vi "Claw Rotation Controller.vi"(8 "error in":errorcluster) -> ()   [LabVIEW 2017]
doc: "This VI executes continuously carrying out the current operation and responding to updates or new operations. It will often contain the timing or control code that is difficult to place directly in TeleOp. This VI generally opens all sensors and motors and isolates the rest of the robot code from knowing how the operations are carried out."
uses:
  Claw Rotation Setpoints.ctl
  Claw Rotation Operations.ctl
  Users/Public/Documents/Cross The Road Electronics/Phoenix-LabVIEW/Motor Controller/Controls/CTRE_Phoenix_MotorControl_ControlMode.ctl
  <vilib>/Rock Robotics/WPI/ThirdParty/Phoenix-LabVIEW/Motor Controller/Controls/CTRE_Phoenix_MotorControl_NeutralMode.ctl
  <vilib>/Rock Robotics/SystemInterfaces/DIO/FPGA_DIOChannel.ctl
  <vilib>/addons/control/pid/pid.llb/PID (DBL).vi
  <vilib>/addons/control/pid/NI_PID_pid.lvlib
  <vilib>/Rock Robotics/Network Tables/NT Write Boolean.vi
panel:
  out "Current\nCmd":string
  # "Tip: It may be helpful to observe inputs and sensor values.\nYou may also want to display tuning or debugging controls."
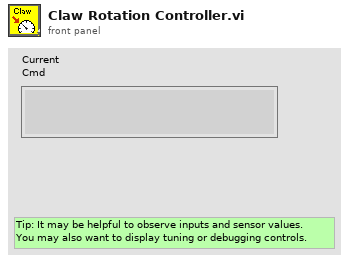
[diagram p1: front panel]
types:
  T1 = typedef "FPGA_DIOChannel.ctl" = enum8{"DIO 0", "DIO 1", "DIO 2", "DIO 3", "DIO 4", "DIO 5", "DIO 6", "DIO 7", "DIO 8", "DIO 9", "DIO MXP 0", "DIO MXP 1", "DIO MXP 2", "DIO MXP 3", "DIO MXP 4", "DIO MXP 5", "DIO MXP 6", "DIO MXP 7", "DIO MXP 8", "DIO MXP 9", "DIO MXP 10", "DIO MXP 11", "DIO MXP 12", "DIO MXP 13", "DIO MXP 14", "DIO MXP 15", "SPI Port CS1", "SPI Port CS2", "SPI Port CS3", "SPI Port MISO", "SPI Port MOSI", "Invalid"}
  T2 = typedef "CTRE_Phoenix_MotorControl_ControlMode.ctl" = u16
  T3 = typedef "CTRE_Phoenix_MotorControl_NeutralMode.ctl" = enum8{"EEPROMSetting", "Override to Coast", "Override to Brake"}
  T4 = typedef "Claw Rotation Setpoints.ctl" = cluster{"Operation":T5, "Setpoint":dbl, "Duration":dbl}
  T5 = typedef "Claw Rotation Operations.ctl" = enum16{"Reserve", "Read Current", "Immediate", "Rotate Manual", "Preset Position"}
  T6 = typedef "WPI_MotorControlDeviceRef.ctl" = cluster{"DeviceStatus":errorcluster, "Type":T7, "PWM":cluster{"PWM Channel":T8, "DeadBand":T9}, "CAN":cluster{"Device Number":u8, "SetOutput VI Ref":variant, "GetOutput VI Ref":variant, "Enable VI Ref":variant, "Disable VI Ref":variant, "Data":variant}, "Invert":bool, "DIO PWM":cluster{"PWM \"Enable\" Channel":T8, "DIOChannel":T1, "PWM Rate":dbl}}
  T7 = typedef "WPI_MotorControlType.ctl" = enum16{"PWM", "CAN", "DIO PWM"}
  T8 = typedef "FPGA_DIOPWMChannel.ctl" = enum8{"PWM 0", "PWM 1", "PWM 2", "PWM 3", "PWM 4", "PWM 5", "PWM 6", "PWM 7", "PWM 8", "PWM 9", "PWM MXP 0", "PWM MXP 1", "PWM MXP 2", "PWM MXP 3", "PWM MXP 4", "PWM MXP 5", "PWM MXP 6", "PWM MXP 7", "PWM MXP 8", "PWM MXP 9", "Invalid"}
  T9 = typedef "WPI_PWMDeadband.ctl" = cluster{"Name":string, "maxPositivePwm":i32, "minPositivePwm":i32, "centerPwm":i32, "maxNegativePwm":i32, "minNegativePwm":i32, "angularRange":u16}
  T10 = typedef "WPI_DigitalInputDevRef.ctl" = cluster{"DevStatus":errorcluster, "DIO Channel":T1}
  T11 = typedef "Command Status Info.ctl" = cluster{"Name":string, "Status":T12, "notifier out":T13}
  T12 = typedef "Completion Status.ctl" = enum16{"Successful", "Aborted", "Incomplete"}
  T13 = typedef "Completion Notifier.ctl" = refnum<notifier>
  T14 = cluster{"Current Command":T4, "Command Timing":cluster{"Start Time (ms)":u32, "Iterations":i32}, "Command Arguments":cluster{"Command Info":T11, "Description":string, "Default Command":T4, "queue out":refnum<queue>, "Subsystem Name":string}}
  T15 = cluster{"proportional gain (Kc)":dbl, "integral time (Ti, min)":dbl, "derivative time (Td, min)":dbl}
  T16 = typedef "WPI_AnalogChannelDevRef.ctl" = cluster{"DevStatus":errorcluster, "Analog Channel":T17}
  T17 = typedef "FPGA_AIChannel.ctl" = enum8{"AI 0", "AI 1", "AI 2", "AI 3", "AI MXP 0", "AI MXP 1", "AI MXP 2", "AI MXP 3", "Invalid"}
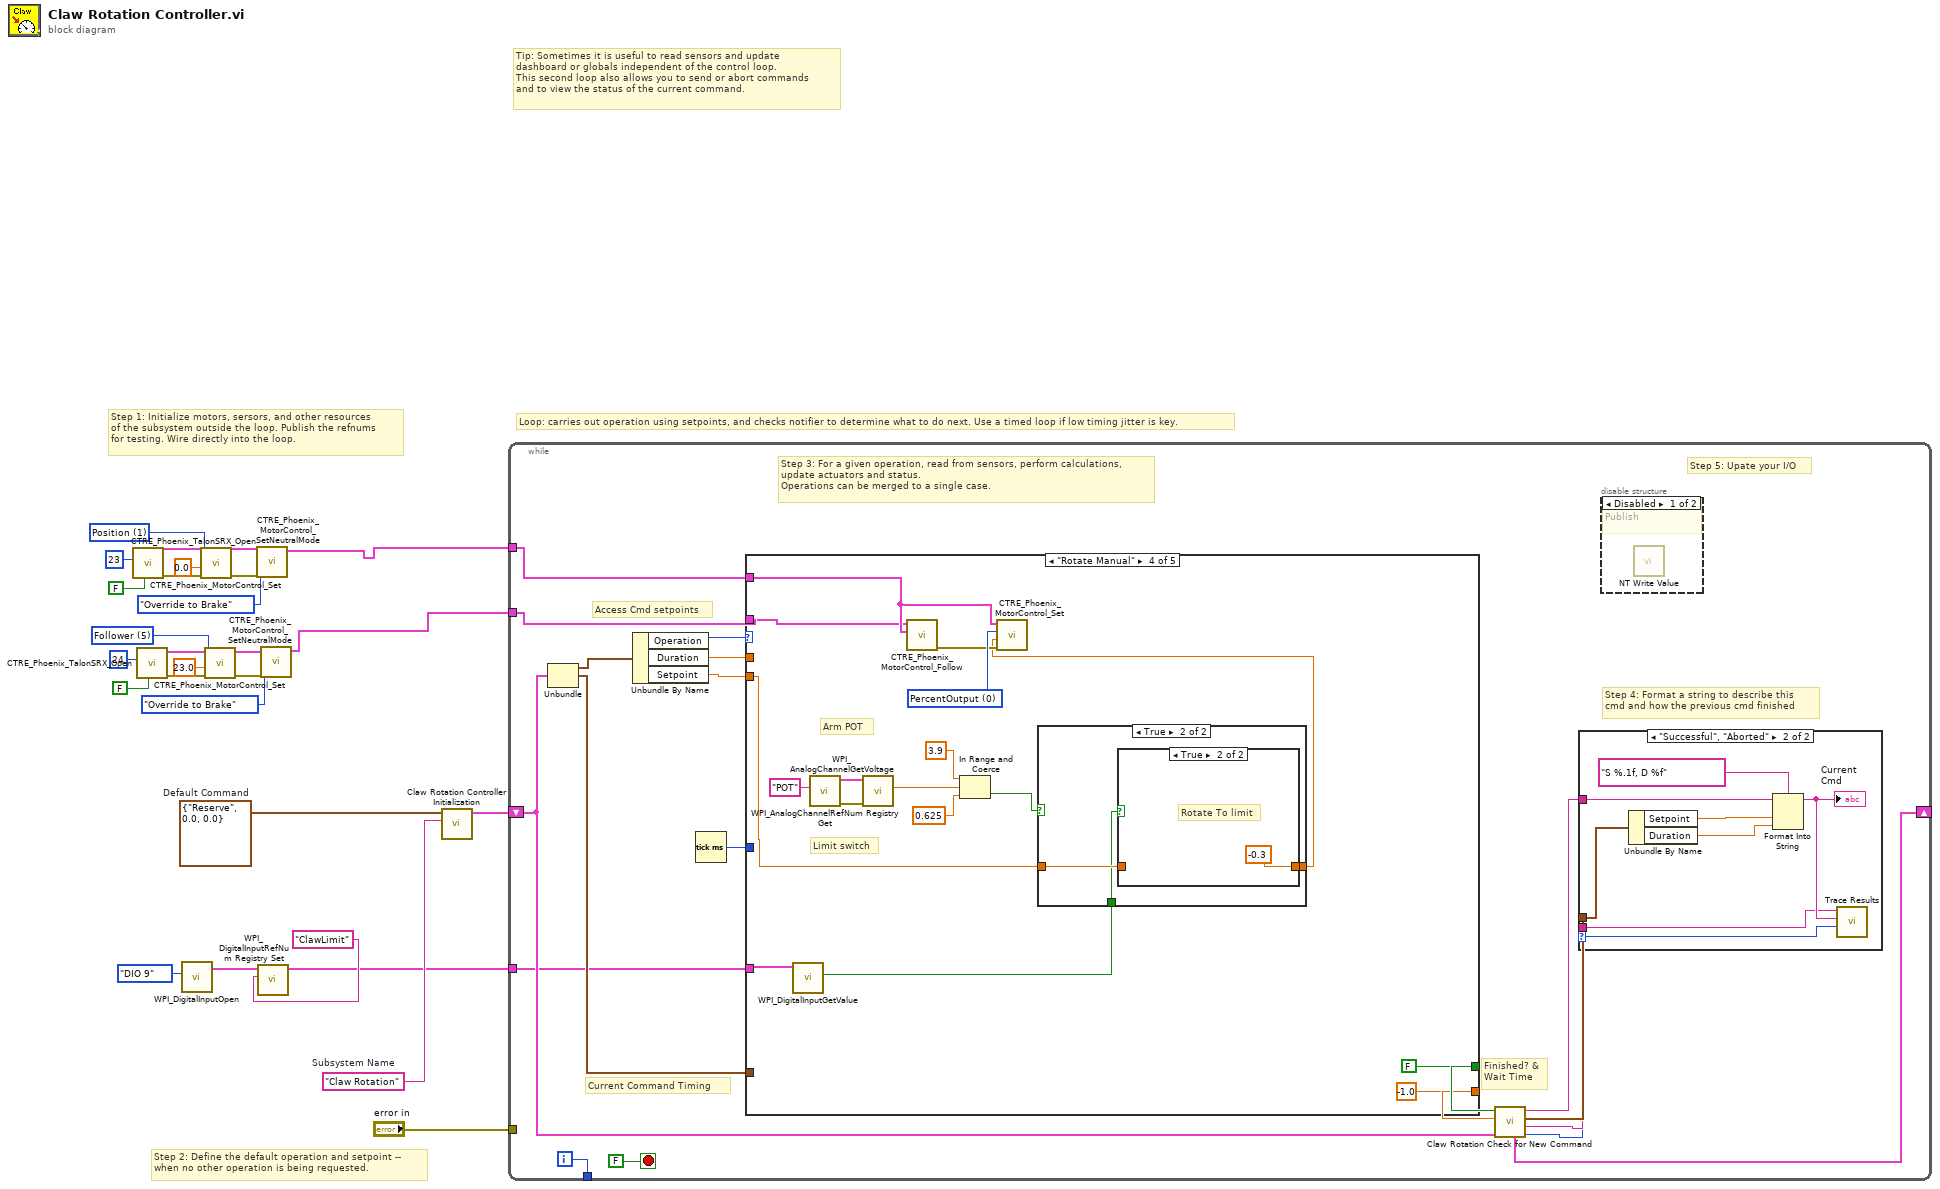
[diagram p0: block diagram]
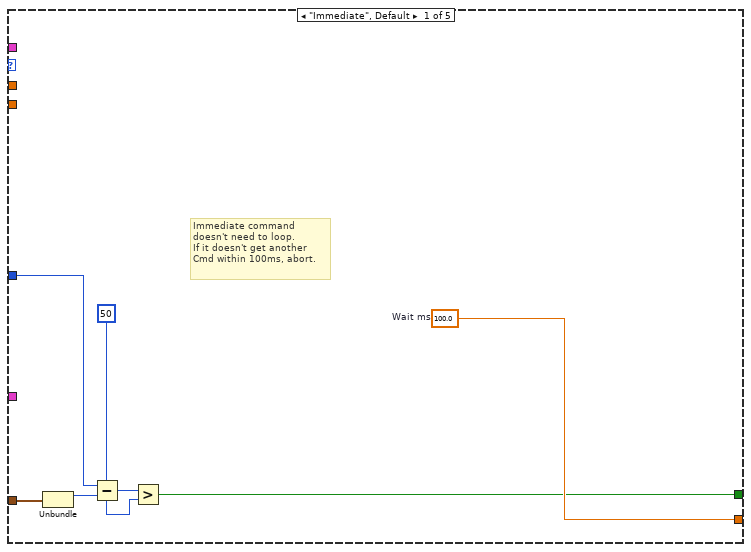
[diagram p4: hidden frame]
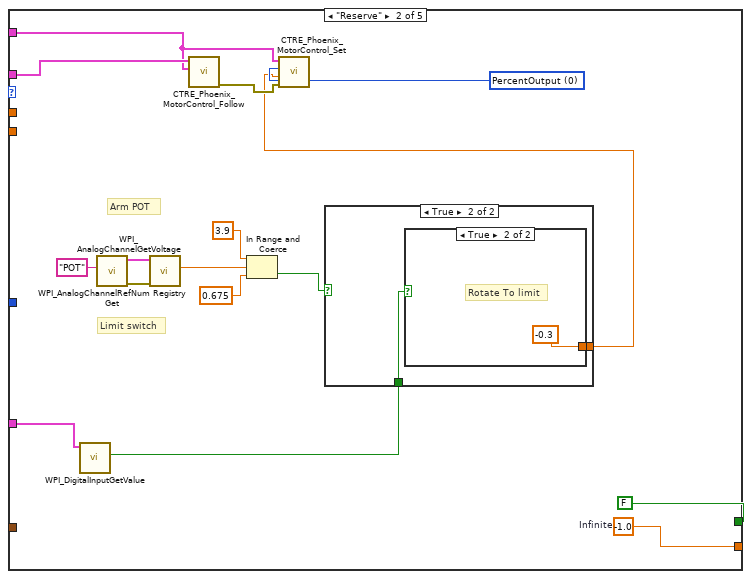
[diagram p5: hidden frame]
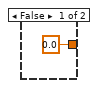
[diagram p6: hidden frame]
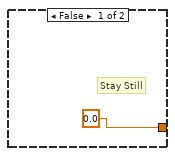
[diagram p7: hidden frame]
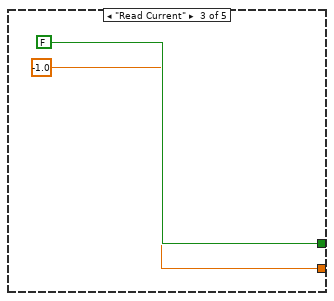
[diagram p8: hidden frame]
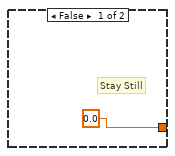
[diagram p10: hidden frame]
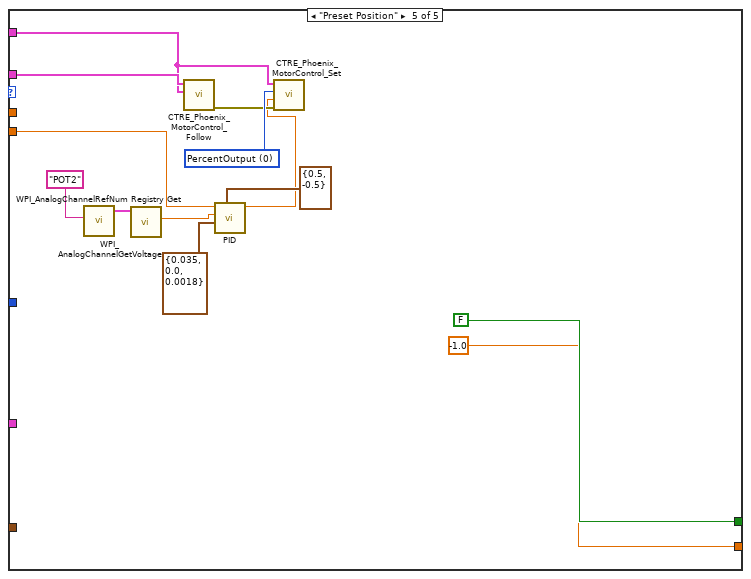
[diagram p11: hidden frame]
diagram:
  w10 = T2 5 items=["PercentOutput"=0, "Position"=1, "Velocity"=2, "Current"=3, "Follower"=5, "MotionProfile"=6, "MotionMagic"=7, "MotionMagicArc"=8, "MotionProfileArc"=10, "Disabled"=15] ("Control Mode")
  w19 = T2 1 items=["PercentOutput"=0, "Position"=1, "Velocity"=2, "Current"=3, "Follower"=5, "MotionProfile"=6, "MotionMagic"=7, "MotionMagicArc"=8, "MotionProfileArc"=10, "Disabled"=15] ("Control Mode")
  w25 = T4 {"Operation"=enum."Reserve", "Setpoint"=0.0, "Duration"=0.0}  # Default Command
  w26 = "Claw Rotation"  # Subsystem Name
  # "Tip: Sometimes it is useful to read sensors and update\ndashboard or globals independent of the control loop.\nThis second loop also allows you to send or abort commands\nand to view the status of the current command."
  # "Step 2: Define the default operation and setpoint --\nwhen no other operation is being requested."
  # "Step 1: Initialize motors, sersors, and other resources\nof the subsystem outside the loop. Publish the refnums\nfor testing. Wire directly into the loop."
  # "Loop: carries out operation using setpoints, and checks notifier to determine what to do next. Use a timed loop if low timing jitter is key."
  n1 = call <vilib>:"CTRE_Phoenix_TalonSRX_Open.vi"("Invert"=FALSE, "Device Number"=u8 23) -> ("error out"=w22:errorcluster, "CAN Talon SRX Ref"=w21:T6)  [unwired: 8 in]
  n2 = call <vilib>:"CTRE_Phoenix_TalonSRX_Open.vi"("Invert"=FALSE, "Device Number"=u8 24) -> ("error out"=w13:errorcluster, "CAN Talon SRX Ref"=w12:T6)  [unwired: 8 in]
  n3 = call <vilib>:"WPI_DigitalInputOpen.vi"("DIO Channel"=FPGA_DIOChannel."DIO 9") -> ("DigitalInputDevRef"=w6:T10)  [unwired: 9 in, 1 out]
  n4 = call <vilib>:"CTRE_Phoenix_MotorControl_Set.vi"("error in (no error)"=w22, "Output"=0.0, "Control Mode"=w19, "PhoenixMotorControlDevRef"=w21) -> ("error out"=w24:errorcluster, "PhoenixMotorControlDevRef"=w23:T6)  [unwired: 6 in]
  n5 = call <vilib>:"CTRE_Phoenix_MotorControl_Set.vi"("error in (no error)"=w13, "Output"=23.0, "Control Mode"=w10, "PhoenixMotorControlDevRef"=w12) -> ("error out"=w15:errorcluster, "PhoenixMotorControlDevRef"=w14:T6)  [unwired: 6 in]
  n6 = call <vilib>:"CTRE_Phoenix_MotorControl_SetNeutralMode.vi"("error in (no error)"=w24, "Motor Control Neutral Mode"=CTRE_Phoenix_MotorControl_NeutralMode."Override to Brake", "PhoenixMotorControlDevRef"=w23) -> ("PhoenixMotorControlDevRef"=w1:T6)  [unwired: 7 in, 1 out]
  n7 = call <vilib>:"WPI_DigitalInputRefNum Registry Set.vi"("refnum name"="ClawLimit", "DigitalInputDevRef"=w6) -> ("DigitalInputDevRef"=w3:T10)  [unwired: 8 in, 1 out]
  n8 = call <vilib>:"CTRE_Phoenix_MotorControl_SetNeutralMode.vi"("error in (no error)"=w15, "Motor Control Neutral Mode"=CTRE_Phoenix_MotorControl_NeutralMode."Override to Brake", "PhoenixMotorControlDevRef"=w14) -> ("PhoenixMotorControlDevRef"=w2:T6)  [unwired: 7 in, 1 out]
  n9 = call "Claw Rotation Controller Initialization.vi"("Subsystem Name"=w26, "Default Command"=w25) -> ("Current Command"=w27:T14)  [unwired: 9 in]
  n10 = while {
    shift-right: [w39] -> _
    shift-left: w27 -> [w32]
    tunnel: [w46] -> _
    tunnel: "error in" -> [_]
    tunnel: w1 -> [w31]
    tunnel: w2 -> [w30]
    tunnel: w3 -> [w29]
    i -> [w46]
    stop <- FALSE stop-if-true
    # "Step 5: Upate your I/O"
    # "Step 4: Format a string to describe this\ncmd and how the previous cmd finished"
    # "Current Command Timing"
    # "Access Cmd setpoints"
    # "Finished? &\nWait Time"
    # "Step 3: For a given operation, read from sensors, perform calculations,\nupdate actuators and status.\nOperations can be merged to a single case."
    n11 = Unbundle(w32) -> ("Current Command"=w45:T4, "Command Timing"=w41:cluster{"Start Time (ms)":u32, "Iterations":i32})  [unwired: 1 out]
    n12 = Unbundle By Name(w45) -> ("Operation"=w44:T5, "Duration"=w43:dbl, "Setpoint"=w40:dbl)
    n13 = Tick Count (ms)() -> (millisecond timer value=w42:u32)
    n14 = case shown="\"Rotate Manual\"" w44 {
      tunnel: [w62 w78 -1.0 ("Infinite") -1.0 ("Infinite") -1.0 ("Infinite")] -> w37
      tunnel: [w56 FALSE ("ignore previous (F)") FALSE ("ignore previous (F)") FALSE ("ignore previous (F)") FALSE ("ignore previous (F)")] -> w38
      tunnel: w41 -> [w58 _ _ _ _]
      tunnel: w43 -> [_ _ _ _ _]
      tunnel: w42 -> [w57 _ _ _ _]
      tunnel: w40 -> [_ _ _ w90 w112]
      tunnel: w31 -> [_ w63 _ w99 w116]
      tunnel: w30 -> [_ w64 _ w86 w118]
      tunnel: w29 -> [_ w66 _ w88 _]
      frame "Immediate", Default {
        w62 = 100.0  # Wait ms
        # "Immediate command\ndoesn't need to loop.\nIf it doesn't get another\nCmd within 100ms, abort."
        n15 = Unbundle(w58) -> ("Start Time (ms)"=w61:u32)  [unwired: 1 out]
        n16 = Subtract(x=w57, y=w61) -> (x-y=w60:u32)
        n17 = Greater?(x=w60, y=u8 50 ("Left Motor")) -> (0:w56:bool)
      }
      frame "Reserve" {
        w76 = T2 0 items=["PercentOutput"=0, "Position"=1, "Velocity"=2, "Current"=3, "Follower"=5, "MotionProfile"=6, "MotionMagic"=7, "MotionMagicArc"=8, "MotionProfileArc"=10, "Disabled"=15] ("Control Mode")
        w78 = -1.0  # Infinite
        # "Arm POT"
        # "Limit switch"
        n18 = call <vilib>:"WPI_DigitalInputGetValue.vi"("DigitalInputDevRef"=w66) -> ("Value"=w67:bool)  [unwired: 8 in, 2 out]
        n19 = call <vilib>:"WPI_AnalogChannelRefNum Registry Get.vi"("refnum name"="POT") -> ("error out"=w74:errorcluster, "AIDeviceRef"=w73:T16)  [unwired: 9 in]
        n20 = call <vilib>:"WPI_AnalogChannelGetVoltage.vi"("error in (no error)"=w74, "AIDeviceRef"=w73) -> ("Voltage"=w71:dbl)  [unwired: 7 in, 2 out]
        n21 = call <vilib>:"CTRE_Phoenix_MotorControl_Follow.vi"("Master Controller to Follow"=w63, "PhoenixMotorControlDevRef"=w64) -> ("error out"=w75:errorcluster)  [unwired: 8 in, 1 out]
        n22 = In Range and Coerce(upper limit=3.9, x=w71, lower limit=0.675) -> (In Range?=w68:bool)  [unwired: 1 out]
        n23 = case shown="True" w68 {
          tunnel: [0.0 w81] -> w65
          tunnel: w67 -> [_ w80]
          frame False {
          }
          frame True {
            n24 = case shown="True" w80 {
              tunnel: [0.0 -0.3] -> w81
              frame False {
                # "Stay Still"
              }
              frame True {
                # "Rotate To limit"
              }
            }
          }
        }
        n25 = call <vilib>:"CTRE_Phoenix_MotorControl_Set.vi"("error in (no error)"=w75, "Output"=w65, "Control Mode"=w76, "PhoenixMotorControlDevRef"=w63) -> ()  [unwired: 6 in, 2 out]
      }
      frame "Read Current" {
      }
      frame "Rotate Manual" {
        w100 = T2 0 items=["PercentOutput"=0, "Position"=1, "Velocity"=2, "Current"=3, "Follower"=5, "MotionProfile"=6, "MotionMagic"=7, "MotionMagicArc"=8, "MotionProfileArc"=10, "Disabled"=15] ("Control Mode")
        # "Arm POT"
        # "Limit switch"
        n26 = call <vilib>:"WPI_DigitalInputGetValue.vi"("DigitalInputDevRef"=w88) -> ("Value"=w87:bool)  [unwired: 8 in, 2 out]
        n27 = call <vilib>:"WPI_AnalogChannelRefNum Registry Get.vi"("refnum name"="POT") -> ("error out"=w97:errorcluster, "AIDeviceRef"=w96:T16)  [unwired: 9 in]
        n28 = call <vilib>:"WPI_AnalogChannelGetVoltage.vi"("error in (no error)"=w97, "AIDeviceRef"=w96) -> ("Voltage"=w94:dbl)  [unwired: 7 in, 2 out]
        n29 = call <vilib>:"CTRE_Phoenix_MotorControl_Follow.vi"("Master Controller to Follow"=w99, "PhoenixMotorControlDevRef"=w86) -> ("error out"=w98:errorcluster)  [unwired: 8 in, 1 out]
        n30 = In Range and Coerce(upper limit=3.9, x=w94, lower limit=0.625) -> (In Range?=w91:bool)  [unwired: 1 out]
        n31 = case shown="True" w91 {
          tunnel: w90 -> [w103 w106]
          tunnel: [w103 w105] -> w89
          tunnel: w87 -> [_ w104]
          frame False {
          }
          frame True {
            n32 = case shown="True" w104 {
              tunnel: w106 -> [_ _]
              tunnel: [0.0 -0.3] -> w105
              frame False {
                # "Stay Still"
              }
              frame True {
                # "Rotate To limit"
              }
            }
          }
        }
        n33 = call <vilib>:"CTRE_Phoenix_MotorControl_Set.vi"("error in (no error)"=w98, "Output"=w89, "Control Mode"=w100, "PhoenixMotorControlDevRef"=w99) -> ()  [unwired: 6 in, 2 out]
      }
      frame "Preset Position" {
        w119 = T2 0 items=["PercentOutput"=0, "Position"=1, "Velocity"=2, "Current"=3, "Follower"=5, "MotionProfile"=6, "MotionMagic"=7, "MotionMagicArc"=8, "MotionProfileArc"=10, "Disabled"=15] ("Control Mode")
        n34 = call <vilib>:"WPI_AnalogChannelRefNum Registry Get.vi"("refnum name"="POT2") -> ("AIDeviceRef"=w115:T16)  [unwired: 9 in, 1 out]
        n35 = call <vilib>:"WPI_AnalogChannelGetVoltage.vi"("AIDeviceRef"=w115) -> ("Voltage"=w113:dbl)  [unwired: 8 in, 2 out]
        n36 = call <vilib>:"CTRE_Phoenix_MotorControl_Follow.vi"("Master Controller to Follow"=w116, "PhoenixMotorControlDevRef"=w118) -> ("error out"=w117:errorcluster)  [unwired: 8 in, 1 out]
        n37 = call-poly <vilib>:"PID.vi"("output range"=cluster{"output high":dbl, "output low":dbl} {"output high"=0.5, "output low"=-0.5}, "PID gains"=T15 {"proportional gain (Kc)"=0.035, "integral time (Ti, min)"=0.0, "derivative time (Td, min)"=0.0018}, "process variable"=w113, "setpoint"=w112) -> ("output"=w109:dbl)  [unwired: 6 in, 1 out]
        n38 = call <vilib>:"CTRE_Phoenix_MotorControl_Set.vi"("error in (no error)"=w117, "Output"=w109, "Control Mode"=w119, "PhoenixMotorControlDevRef"=w116) -> ()  [unwired: 6 in, 2 out]
      }
    }
    n39 = call "Claw Rotation Check for New Command.vi"("Current Command"=w32, "Wait time (ms)"=w37, "Finished?"=w38) -> ("Completion"=w33:T12, "Subsystem Name"=w34:string, "Current Command"=w35:T4, "Initial Trace String"=w36:string, "NextCommand"=w39:T14)  [unwired: 4 in]
    n40 = case shown="\"Successful\", \"Aborted\"" w33 {
      selector: w33 -> [_ w55]
      tunnel: w36 -> [_ w51]
      tunnel: w35 -> [_ w52]
      tunnel: w34 -> [_ w48]
      frame "Incomplete", Default {
        # "Continuing current command"
      }
      frame "Successful", "Aborted" {
        # "Report and setup for next command"
        n41 = Unbundle By Name(w52) -> ("Setpoint"=w54:dbl, "Duration"=w49:dbl)
        n42 = Format Into String(format string="S %.1f, D %f", initial string=w51, w54, w49) -> (resulting string=w50:string)  [unwired: 1 in, 1 out]
        "Current\nCmd" <- w50
        n43 = call <vilib>:"Trace Results.vi"("Status of previous command"=w55, "Description"=w50, "Subsystem"=w48) -> ()  [unwired: 9 in]
      }
    }
    n44 = disable-structure shown="Disabled" {
      frame Disabled {
        # "Publish"
        n45 = call-poly <vilib>:"NT Write Value.vi"() -> ()  [unwired: 11 in, 1 out]
      }
      frame Enabled {
      }
    }
  }
